vi "initialize.vi"(0 "HGF_FGV_Subset":refnum<class "HGF_FGV_SubSet.lvclass">, 3 "initializationData":variant, 5 "error in (no error)":errorcluster, 7 "binaryString":string, 8 "I8 Array":i8[](array[numeric]), 9 "prependSize? (T)":bool, 11 "byteOrder (0:big-endian, network order)":T1(ring)) -> (14 "dup HGF_FGV_Subset":refnum<class "HGF_FGV_SubSet.lvclass">, 17 "found?":bool, 19 "error out":errorcluster)   [LabVIEW 2012, in "HGF_FGV.lvlib" / "HGF_FGV_SubSet.lvclass"]
doc: "This is a dynamic dispatch VI to be implemented by child classes to initialize their attributes.\n\n<B>Attention:</B> Support for Variant for initialization data only."
uses:
  HGF_FGV_SubSet.lvclass
  HGF_FGV_Action/HGF_FGV_Action.lvclass
  HGF_FGV_SubSet.lvclass/HGF_FGV_SubSet.ctl
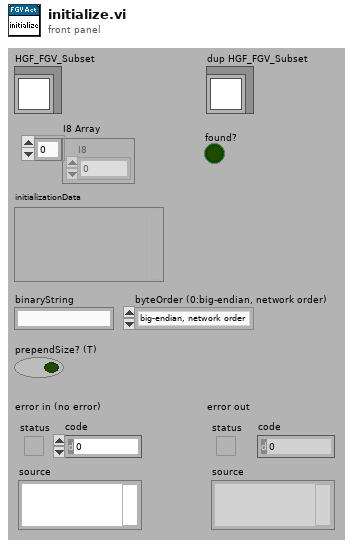
[diagram p1: front panel]
types:
  T1 = enum16{"big-endian, network order", "native, host order", "little-endian"}
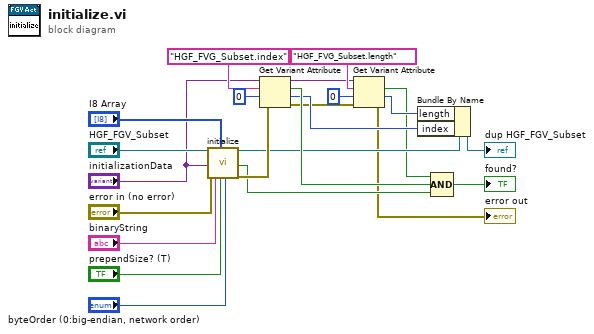
[diagram p0: block diagram]
diagram:
  n1 = call-parent "initialize.vi"("HGF_Factory"="HGF_FGV_Subset", "initializationData"="initializationData", "error in (no error)"="error in (no error)", "binaryString"="binaryString", "I8 Array"="I8 Array", "prependSize? (T)"="prependSize? (T)", "byteOrder (0:big-endian, network order)"="byteOrder (0:big-endian, network order)") -> ("dup HGF_Factory"=w13:refnum<class "HGF_FGV_SubSet.lvclass">, "found?"=w19:bool, "error out"=w20:errorcluster)  [unwired: 1 in, 9 out]
  n2 = Get Variant Attribute(Variant="initializationData", name="HGF_FVG_Subset.index", default value (empty Variant)=u32 0, error in=w20) -> (duplicate Variant=w9:variant, found=w14:bool, value=w12:u32, error out=w5:errorcluster)
  n3 = Get Variant Attribute(Variant=w9, name="HGF_FVG_Subset.length", default value (empty Variant)=u32 0, error in=w5) -> (found=w6:bool, value=w7:u32, error out=→"error out":errorcluster)  [unwired: 1 out]
  n4 = Bundle By Name(cluster=w13, "length"=w7, "index"=w12) -> (→"dup HGF_FGV_Subset":refnum<class "HGF_FGV_SubSet.lvclass">)
  n5 = Compound Arithmetic op=AND(w6, w14, w19) -> (→"found?":bool)
